vi "Whileloops.vi"() -> ()   [LabVIEW 2014]
panel:
  out "Current Number":dbl format="%#.0f"
  out "Number of Iterations":i32
  in  "Number to Match":dbl=50.0 min=0.0 max=1000.0 step=1.0 format="%#.0f"
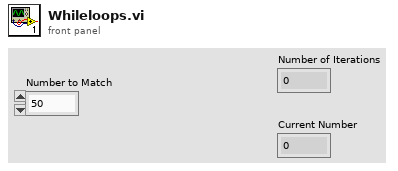
[diagram p1: front panel]
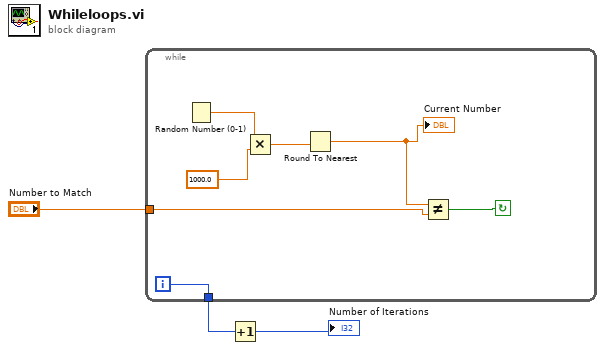
[diagram p0: block diagram]
diagram:
  n1 = while {
    tunnel: [w10] -> w2
    tunnel: "Number to Match" -> [w8]
    i -> [w10]
    stop <- w9 continue-if-true
    n2 = Random Number (0-1)() -> (number: 0 to 1=w6:dbl)
    n3 = Multiply(x=w6, y=1000.0 ("x*y")) -> (x*y=w5:dbl)
    n4 = Round To Nearest(number=w5) -> (nearest integer value=w4:dbl)
    "Current Number" <- w4
    n5 = Not Equal?(x=w4, y=w8) -> (x != y?=w9:bool)
  }
  n6 = Increment(x=w2) -> (x+1=→"Number of Iterations":i32)
